vi "Insert Value[] (Value).vi"(7 "key":string[](array[string]), 8 "error in (no error)":errorcluster, 10 "JSON Value in":refnum<class "JSON Value.lvclass">, 11 "JSON Value in":refnum<class "JSON Value.lvclass">) -> (0 "error out":errorcluster, 1 "replaced":bool, 3 "JSON Value out":refnum<class "JSON Value.lvclass">)   [LabVIEW 2016, in "JSON Value.lvclass"]
uses:
  JSON Value.lvclass
  Insert Value (Value).vi
  Array/Replace Array Subset/Replace Array Subset (Value).vi
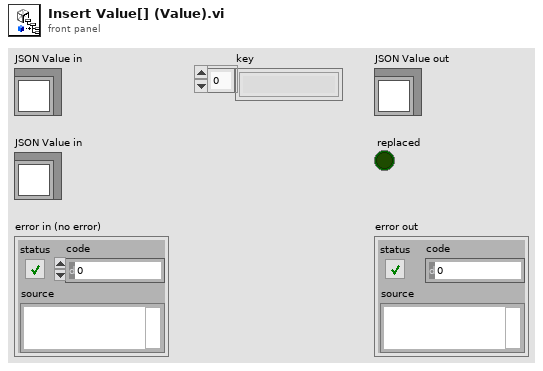
[diagram p1: front panel]
types:
  T1 = typedef "JSON Value.lvclass/JSON Types.ctl" = enum16{"String", "Numeric", "Boolean", "NULL", "Object", "Array"}
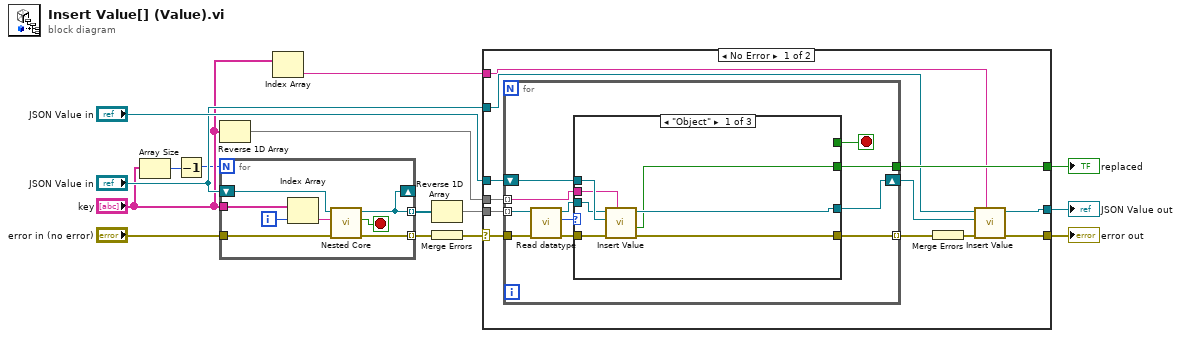
[diagram p0: block diagram]
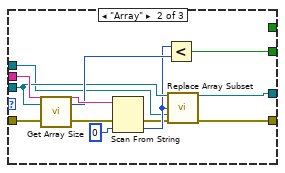
[diagram p2: hidden frame]
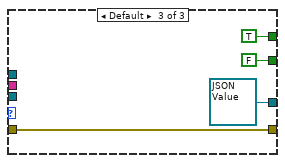
[diagram p3: hidden frame]
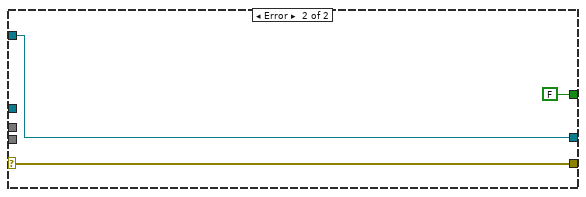
[diagram p4: hidden frame]
diagram:
  n1 = Array Size(array="key") -> (size(s)=w3:i32)
  n2 = Decrement(x=w3) -> (x-1=w4:i32)
  n3 = Reverse 1D Array(array="key") -> (reversed array=w12:string[])
  n4 = for {
    N: w4 -> [_]
    tunnel: "key" -> [w19]
    shift-right: [w16] -> _
    shift-left: "JSON Value in" -> [w23]
    tunnel: "error in (no error)" -> [w22]
    tunnel: [w21] -> w11 mode=indexing
    tunnel: [w16] -> w2 mode=indexing
    i -> [w18]
    stop <- w20 stop-if-true
    n5 = Index Array(array=w19, index=w18) -> (element=w17:string)
    n6 = call "Nested Core.vi"("error in (no error)"=w22, "key"=w17, "JSON Value in"=w23) -> ("error out"=w21:errorcluster, "stop?"=w20:bool, "JSON Value out"=w16:refnum<class "JSON Value.lvclass">)  [unwired: 6 in]
  }
  n7 = Index Array(array="key") -> (element=w5:string)  [unwired: 1 in]
  n8 = Reverse 1D Array(array=w2) -> (reversed array=w13:refnum<class "JSON Value.lvclass">[])
  n9 = Merge Errors(w11) -> (w1:errorcluster)
  n10 = case shown="No Error" w1 {
    selector: w1 -> [w24 w71]
    tunnel: [w35 FALSE ("replaced")] -> w15
    tunnel: "JSON Value in" -> [w34 _]
    tunnel: w13 -> [w33 _]
    tunnel: w12 -> [w32 _]
    tunnel: "JSON Value in" -> [w31 w70]
    tunnel: [w30 w70] -> w8
    tunnel: [w29 w71] -> w7
    tunnel: w5 -> [w28 _]
    frame No Error {
      n11 = for {
        tunnel: w32 -> [w39] mode=indexing
        tunnel: w24 -> [w44]
        tunnel: [w43] -> w27 mode=indexing
        tunnel: [w40] -> w35
        tunnel: w33 -> [w36] mode=indexing
        shift-right: [w38] -> w26
        shift-left: w34 -> [w37]
        stop <- w41 stop-if-true
        n12 = call "Read datatype.vi"("error in (no error)"=w44, "JSON Datatype in"=w36) -> ("error out"=w42:errorcluster, "datatype"=w45:T1, "JSON Datatype out"=w46:refnum<class "JSON Value.lvclass">)  [unwired: 7 in]
        n13 = case shown="\"Object\"" w45 {
          tunnel: w39 -> [w48 w64 _]
          tunnel: [w50 w61 refnum<class "JSON Value.lvclass"> refnum ("JSON Object in")] -> w38
          tunnel: w46 -> [w47 w60 _]
          tunnel: [w52 w54 w68] -> w43
          tunnel: w42 -> [w53 w57 w68]
          tunnel: [_ _ TRUE] -> w41
          tunnel: [w49 w62 FALSE] -> w40
          tunnel: w37 -> [w51 w58 _]
          frame "Object" {
            n14 = call-poly "Insert Value.vi"("key"=w48, "error in (no error)"=w53, 10:"JSON Value in"=w51, 11:"JSON Value in"=w47) -> ("error out"=w52:errorcluster, "replaced"=w49:bool, "JSON Value out"=w50:refnum<class "JSON Value.lvclass">)  [unwired: 5 in]
          }
          frame "Array" {
            n15 = call "Get Array Size.vi"("error in (no error)"=w57, "JSON Value in"=w60) -> ("error out"=w56:errorcluster, "size(s)"=w63:i32)
            n16 = Scan From String(input string=w64, error in=w56, default 1=0 ("index")) -> (error out=w55:errorcluster, output 1=w59:i32)  [unwired: 2 in, 2 out]
            n17 = Less?(x=w59, y=w63) -> (x < y?=w62:bool)
            n18 = call-poly "Replace Array Subset.vi"("JSON Array"=w60, "index"=w59, "new element/subarray"=w58, "error in"=w55) -> ("output JSON Array"=w61:refnum<class "JSON Value.lvclass">, "error out"=w54:errorcluster)  [unwired: 10 in]
          }
          frame Default {
          }
        }
      }
      n19 = Merge Errors(w27) -> (w25:errorcluster)
      n20 = call-poly "Insert Value.vi"("key"=w28, "error in (no error)"=w25, 10:"JSON Value in"=w26, 11:"JSON Value in"=w31) -> ("error out"=w29:errorcluster, "JSON Value out"=w30:refnum<class "JSON Value.lvclass">)  [unwired: 5 in, 1 out]
    }
    frame Error {
    }
  }
  "replaced" <- w15
  "error out" <- w7
  "JSON Value out" <- w8
